vi "Logging Get At.vi"(1 "Time (ms)":u32, 2 "Log Input":T1[](array[typedef])) -> (0 "Output":T1)   [LabVIEW 2012, in "femtoRoboLib.lvlib"]
uses:
  femtoRoboLib.lvlib
  Controls/Log Entry - Full Block.ctl
  Controls/Log Entry.ctl
  Controls/Log Value Type.ctl
  Controls/Log Value Cluster.ctl
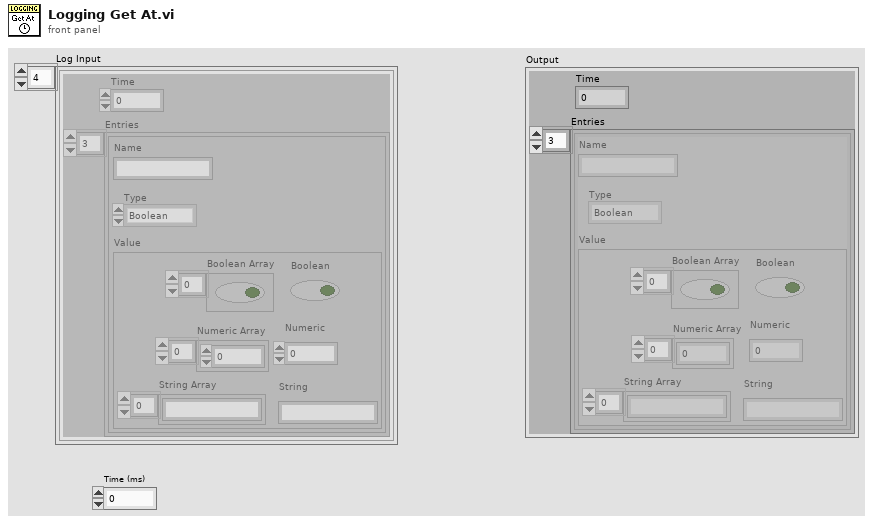
[diagram p1: front panel]
types:
  T1 = typedef "femtoRoboLib.lvlib/Log Entry - Full Block.ctl" = cluster{"Entries":T2[], "Time":u32}
  T2 = typedef "femtoRoboLib.lvlib/Log Entry.ctl" = cluster{"Name":string, "Type":T3, "Value":T4}
  T3 = typedef "femtoRoboLib.lvlib/Log Value Type.ctl" = enum16{"Boolean", "Numeric", "String", "Boolean Array", "Numeric Array", "String Array"}
  T4 = typedef "femtoRoboLib.lvlib/Log Value Cluster.ctl" = cluster{"Boolean Array":bool[], "Boolean":bool, "Numeric Array":dbl[], "Numeric":dbl, "String Array":string[], "String":string}
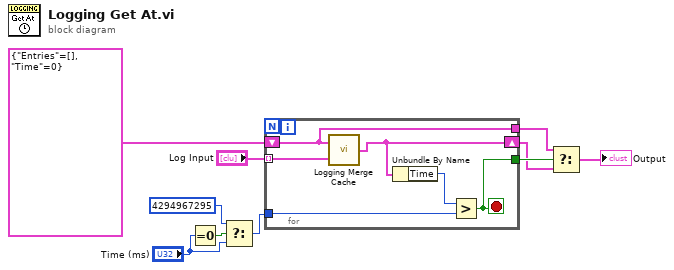
[diagram p0: block diagram]
diagram:
  n1 = Equal To 0?(x="Time (ms)") -> (x = 0?=w8:bool)
  n2 = Select(t=u32 4294967295, s=w8, f="Time (ms)") -> (s? t:f=w5:u32)
  n3 = for {
    shift-right: [w15] -> w1
    shift-left: T1 {"Entries"=[], "Time"=0} ("Cache") -> [w12]
    tunnel: w5 -> [w13]
    tunnel: "Log Input" -> [w14] mode=indexing
    tunnel: [w12] -> w2
    tunnel: [w11] -> w3
    stop <- w11 stop-if-true
    n4 = call "Logging Merge Cache.vi"("Update"=w14, "Cache"=w12) -> ("Output"=w15:T1)
    n5 = Unbundle By Name(w15) -> ("Time"=w16:u32)
    n6 = Greater?(x=w16, y=w13) -> (0:w11:bool)
  }
  n7 = Select(t=w2, s=w3, f=w1) -> (s? t:f=→"Output":T1)
